vi "CamSaturationCheck.vi"(8 "error in (no error)":errorcluster, 11 "Img In":T1) -> (0 "error out":errorcluster, 1 "ImgHist":u32[](graph), 2 "Image Saturated":bool, 3 "Img out":T1)   [LabVIEW 2020]
uses:
  <vilib>/vision/Image Controls.llb/IMAQ Image.ctl
  <vilib>/vision/NI_Vision_Development_Module.lvlib
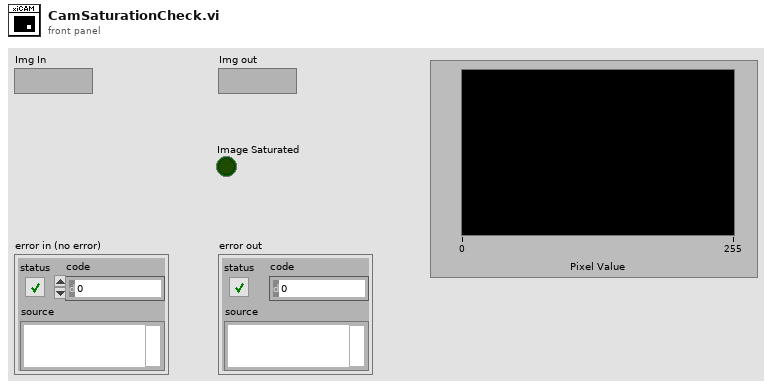
[diagram p1: front panel]
types:
  T1 = typedef "IMAQ Image.ctl" = refnum<image>
  T2 = cluster{"histogram":u32[], "Minimal Value":sgl, "Maximal Value":sgl, "Starting Value":sgl, "Interval Width":sgl, "Mean Value":sgl, "Standard  Variation":sgl, "Area (pixels)":i32}
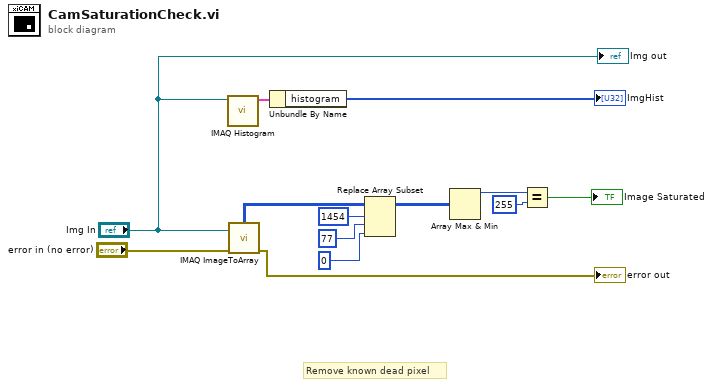
[diagram p0: block diagram]
diagram:
  # "Remove known dead pixel"
  n1 = call "IMAQ Histogram"("Image"="Img In") -> ("Histogram Report"=w10:T2)  [unwired: 9 in, 1 out]
  n2 = call "IMAQ ImageToArray"("error in (no error)"="error in (no error)", "Image"="Img In") -> ("error out"=→"error out":errorcluster, "Image Pixels (U8)"=w8:u8[][])  [unwired: 2 in, 3 out]
  n3 = Unbundle By Name(w10) -> ("histogram"=→"ImgHist":u32[])
  n4 = Replace Array Subset(array=w8, new element=u8 0 ("new element/subarray"), index (row)=1454, index (col)=77 ("disabled index (col)")) -> (w4:u8[][])
  n5 = Array Max & Min(array=w4) -> (max value=w11:u8)  [unwired: 3 out]
  n6 = Equal?(x=w11, y=u8 255) -> (x = y?=→"Image Saturated":bool)
  "Img out" <- "Img In"
